vi "IDN.vi"(11 "uPluggable in":refnum<class "uPluggable.lvclass">) -> (2 "IDN":string)   [LabVIEW 2023, in "uPlug.lvlib" / "uPluggable.lvclass"]
doc: "Type identification string for children classes. \nUsed by plugin-handler to identify the available plugins using mentally recognizable names.\n\nIf not overriden by the child, the default implementation by the abstract parent interface is to use the class name."
uses:
  uPluggable.lvclass
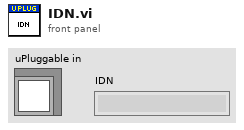
[diagram p1: front panel]
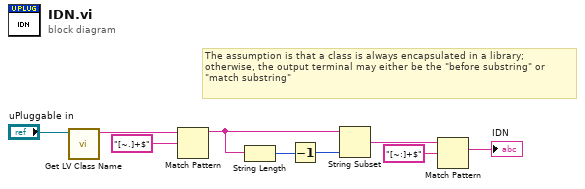
[diagram p0: block diagram]
diagram:
  # "The assumption is that a class is always encapsulated in a library; otherwise, the output terminal may either be the \"before substring\" or \"match substring\""
  n1 = call <vilib>:"Get LV Class Name.vi"("object"="uPluggable in") -> ("class name"=w6:string)  [unwired: 9 in, 1 out]
  n2 = Match Pattern(string=w6, regular expression="[~.]+$") -> (before substring=w3:string)  [unwired: 1 in, 3 out]
  n3 = String Length(string=w3) -> (length=w5:i32)
  n4 = Decrement(x=w5) -> (x-1=w4:i32)
  n5 = String Subset(string=w3, length (rest)=w4) -> (substring=w2:string)  [unwired: 1 in]
  n6 = Match Pattern(string=w2, regular expression="[~:]+$") -> (match substring=→"IDN":string)  [unwired: 1 in, 3 out]
